vi "Get Hopper Current.vi"   [LabVIEW 2016]
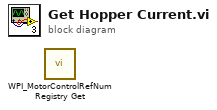
[diagram p0: block diagram]
diagram:
  n1 = call <vilib>:"WPI_MotorControlRefNum Registry Get.vi"() -> ()  [unwired: 10 in, 2 out]
